vi "Finish.vi"   [LabVIEW 2016]
doc: "This VI is called just before exiting. It is expected to close I/O refnum, save collected data, etc."
uses:
  <vilib>/Rock Robotics/WPI/Utilities/WPI_GetSetVariantRefNum.vi
types:
  T1 = typedef "WPI_ServoDeviceRef.ctl" = cluster{"DeviceStatus":errorcluster, "PWM Channel":T2, "DeadBand":T3}
  T2 = typedef "FPGA_DIOPWMChannel.ctl" = enum8{"PWM 0", "PWM 1", "PWM 2", "PWM 3", "PWM 4", "PWM 5", "PWM 6", "PWM 7", "PWM 8", "PWM 9", "PWM MXP 0", "PWM MXP 1", "PWM MXP 2", "PWM MXP 3", "PWM MXP 4", "PWM MXP 5", "PWM MXP 6", "PWM MXP 7", "PWM MXP 8", "PWM MXP 9", "Invalid"}
  T3 = typedef "WPI_PWMDeadband.ctl" = cluster{"Name":string, "maxPositivePwm":i32, "minPositivePwm":i32, "centerPwm":i32, "maxNegativePwm":i32, "minNegativePwm":i32, "angularRange":u16}
  T4 = typedef "WPI_SolenoidDevRef.ctl" = cluster{"DevStatus":errorcluster, "Pneumatics Control Module":u8, "Forward Solenoid Channel":T5, "Reverse Solenoid Channel":T5}
  T5 = typedef "WPI_SolenoidChannel.ctl" = enum8{"Solenoid 0", "Solenoid 1", "Solenoid 2", "Solenoid 3", "Solenoid 4", "Solenoid 5", "Solenoid 6", "Solenoid 7", "Invalid"}
  T6 = typedef "WPI_CompressorDevRef.ctl" = cluster{"DevStatus":errorcluster, "Pneumatics Control Module":u8}
  T7 = typedef "WPI_RobotDriveDevRef.ctl" = cluster{"DevStatus":errorcluster, "Motors[]":T8[], "Square Inputs":bool, "Max Output":dbl}
  T8 = typedef "WPI_MotorControlDeviceRef.ctl" = cluster{"DeviceStatus":errorcluster, "Type":T9, "PWM":cluster{"PWM Channel":T2, "DeadBand":T3}, "CAN":cluster{"Device Number":u8, "SetOutput VI Ref":variant, "GetOutput VI Ref":variant, "Enable VI Ref":variant, "Disable VI Ref":variant, "Data":variant}, "Invert":bool}
  T9 = typedef "WPI_MotorControlType.ctl" = enum16{"PWM", "CAN"}
  T10 = typedef "WPI_JoystickDevRef.ctl" = cluster{"Device":T11}
  T11 = typedef "WPI_JoystickDeviceEnum.ctl" = enum16{"USB 0", "USB 1", "USB 2", "USB 3", "USB 4", "USB 5"}
  T12 = typedef "WPI_EncoderDevRef.ctl" = cluster{"DevStatus":errorcluster, "EncoderIndex":T13, "CounterIndex":T14, "DistancePerCount":dbl, "Decoding Type":T15}
  T13 = typedef "FPGA_EncoderIdx.ctl" = enum8{"Enc 0", "Enc 1", "Enc 2", "Enc 3", "Enc 4", "Enc 5", "Enc 6", "Enc 7", "Invalid"}
  T14 = typedef "FPGA_CounterCtrSystemIndex.ctl" = enum8{"Ctr 0", "Ctr 1", "Ctr 2", "Ctr 3", "Ctr 4", "Ctr 5", "Ctr 6", "Ctr 7", "Invalid"}
  T15 = typedef "WPI_EncoderType.ctl" = enum16{"1x", "2x", "4x"}
  T16 = typedef "WPI_AnalogChannelDevRef.ctl" = cluster{"DevStatus":errorcluster, "Analog Channel":T17}
  T17 = typedef "FPGA_AIChannel.ctl" = enum8{"AI 0", "AI 1", "AI 2", "AI 3", "AI MXP 0", "AI MXP 1", "AI MXP 2", "AI MXP 3", "Invalid"}
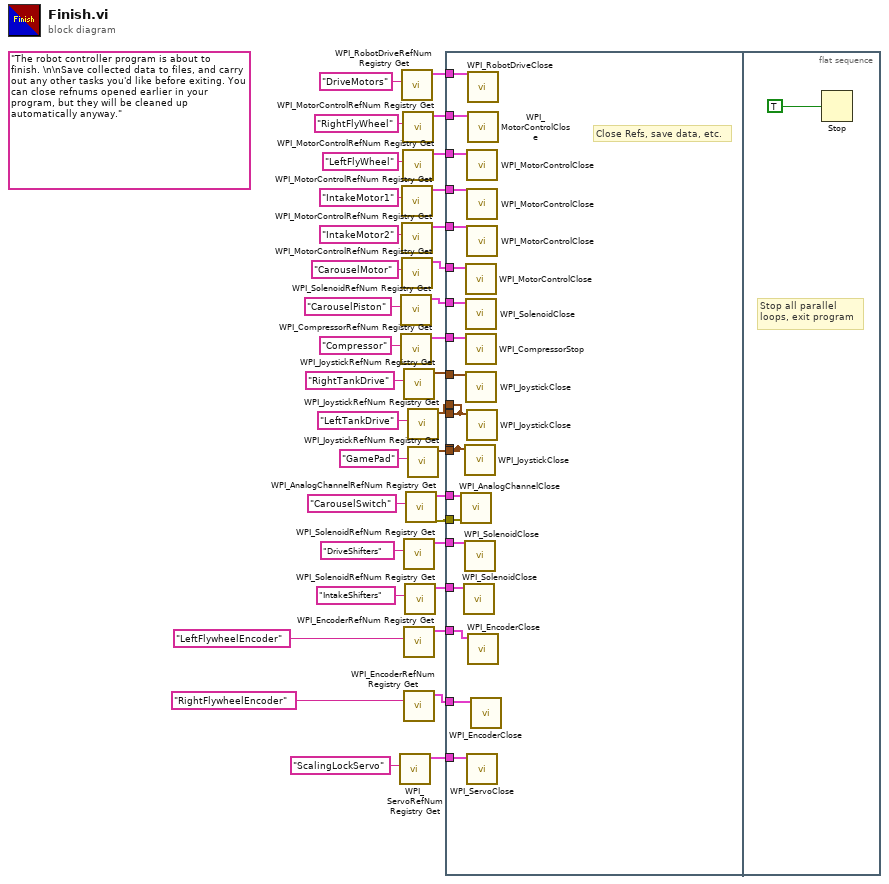
[diagram p0: block diagram]
diagram:
  (unwired) "The robot controller program is about to finish. \n\nSave collected data to files, and carry out any other tasks you'd like before exiting. You can close refnums opened earlier in your program, but they will be cleaned up automatically anyway."
  n1 = call <vilib>:"WPI_ServoRefNum Registry Get.vi"("refnum name"="ScalingLockServo") -> ("ServoDeviceRef"=w2:T1)  [unwired: 9 in, 1 out]
  n2 = call <vilib>:"WPI_SolenoidRefNum Registry Get.vi"("refnum name"="CarouselPiston") -> ("SolenoidDevRef"=w22:T4)  [unwired: 9 in, 1 out]
  n3 = call <vilib>:"WPI_CompressorRefNum Registry Get.vi"("refnum name"="Compressor") -> ("CompressorDevRef"=w21:T6)  [unwired: 9 in, 1 out]
  n4 = call <vilib>:"WPI_RobotDriveRefNum Registry Get.vi"("refnum name"="DriveMotors") -> ("RobotDriveDevRef"=w35:T7)  [unwired: 9 in, 1 out]
  n5 = call <vilib>:"WPI_MotorControlRefNum Registry Get.vi"("refnum name"="IntakeMotor1") -> ("MotorControlDevRef"=w26:T8)  [unwired: 9 in, 1 out]
  n6 = call <vilib>:"WPI_MotorControlRefNum Registry Get.vi"("refnum name"="IntakeMotor2") -> ("MotorControlDevRef"=w25:T8)  [unwired: 9 in, 1 out]
  n7 = call <vilib>:"WPI_MotorControlRefNum Registry Get.vi"("refnum name"="CarouselMotor") -> ("MotorControlDevRef"=w24:T8)  [unwired: 9 in, 1 out]
  n8 = call <vilib>:"WPI_MotorControlRefNum Registry Get.vi"("refnum name"="RightFlyWheel") -> ("MotorControlDevRef"=w28:T8)  [unwired: 9 in, 1 out]
  n9 = call <vilib>:"WPI_MotorControlRefNum Registry Get.vi"("refnum name"="LeftFlyWheel") -> ("MotorControlDevRef"=w27:T8)  [unwired: 9 in, 1 out]
  n10 = call <vilib>:"WPI_JoystickRefNum Registry Get.vi"("refnum name"="RightTankDrive") -> ("JoystickDevRef"=w19:T10)  [unwired: 9 in, 1 out]
  n11 = call <vilib>:"WPI_SolenoidRefNum Registry Get.vi"("refnum name"="DriveShifters") -> ("SolenoidDevRef"=w10:T4)  [unwired: 9 in, 1 out]
  n12 = call <vilib>:"WPI_EncoderRefNum Registry Get.vi"("refnum name"="LeftFlywheelEncoder") -> ("EncoderDevRef"=w3:T12)  [unwired: 9 in, 1 out]
  n13 = call <vilib>:"WPI_EncoderRefNum Registry Get.vi"("refnum name"="RightFlywheelEncoder") -> ("EncoderDevRef"=w4:T12)  [unwired: 9 in, 1 out]
  n14 = call <vilib>:"WPI_SolenoidRefNum Registry Get.vi"("refnum name"="IntakeShifters") -> ("SolenoidDevRef"=w9:T4)  [unwired: 9 in, 1 out]
  n15 = call <vilib>:"WPI_AnalogChannelRefNum Registry Get.vi"("refnum name"="CarouselSwitch") -> ("error out"=w12:errorcluster, "AIDeviceRef"=w11:T16)  [unwired: 9 in]
  n16 = call <vilib>:"WPI_JoystickRefNum Registry Get.vi"("refnum name"="LeftTankDrive") -> ("JoystickDevRef"=w18:T10)  [unwired: 9 in, 1 out]
  n17 = call <vilib>:"WPI_JoystickRefNum Registry Get.vi"("refnum name"="GamePad") -> ("JoystickDevRef"=w17:T10)  [unwired: 9 in, 1 out]
  n18 = flat-sequence {
    tunnel: w35 -> [w53]
    tunnel: w28 -> [w52]
    tunnel: w27 -> [w51]
    tunnel: w26 -> [w50]
    tunnel: w25 -> [w49]
    tunnel: w24 -> [w48]
    tunnel: w22 -> [w47]
    tunnel: w21 -> [w46]
    tunnel: w19 -> [w45]
    tunnel: [w44] -> _
    tunnel: [w43] -> _
    tunnel: w18 -> [w44]
    tunnel: w17 -> [w43]
    tunnel: w12 -> [w42]
    tunnel: w11 -> [w41]
    tunnel: w10 -> [w40]
    tunnel: w9 -> [w39]
    tunnel: w4 -> [w38]
    tunnel: w3 -> [w37]
    tunnel: w2 -> [w36]
    frame #0 {
      # "Close Refs, save data, etc."
      n19 = call <vilib>:"WPI_AnalogChannelClose.vi"("error in (no error)"=w42, "AIDeviceRef"=w41) -> ()  [unwired: 9 in, 1 out]
      n20 = call <vilib>:"WPI_SolenoidClose.vi"("SolenoidDevRef"=w39) -> ()  [unwired: 10 in, 1 out]
      n21 = call <vilib>:"WPI_JoystickClose.vi"("JoystickDevRef"=w43) -> ()  [unwired: 11 in]
      n22 = call <vilib>:"WPI_SolenoidClose.vi"("SolenoidDevRef"=w40) -> ()  [unwired: 10 in, 1 out]
      n23 = call <vilib>:"WPI_MotorControlClose.vi"("MotorControlDevRef"=w48) -> ()  [unwired: 10 in, 1 out]
      n24 = call <vilib>:"WPI_SolenoidClose.vi"("SolenoidDevRef"=w47) -> ()  [unwired: 10 in, 1 out]
      n25 = call <vilib>:"WPI_CompressorStop.vi"("CompressorDevRef"=w46) -> ()  [unwired: 9 in, 2 out]
      n26 = call <vilib>:"WPI_JoystickClose.vi"("JoystickDevRef"=w45) -> ()  [unwired: 11 in]
      n27 = call <vilib>:"WPI_MotorControlClose.vi"("MotorControlDevRef"=w51) -> ()  [unwired: 10 in, 1 out]
      n28 = call <vilib>:"WPI_MotorControlClose.vi"("MotorControlDevRef"=w50) -> ()  [unwired: 10 in, 1 out]
      n29 = call <vilib>:"WPI_MotorControlClose.vi"("MotorControlDevRef"=w49) -> ()  [unwired: 10 in, 1 out]
      n30 = call <vilib>:"WPI_JoystickClose.vi"("JoystickDevRef"=w44) -> ()  [unwired: 11 in]
      n31 = call <vilib>:"WPI_ServoClose.vi"("ServoDeviceRef"=w36) -> ()  [unwired: 10 in, 1 out]
      n32 = call <vilib>:"WPI_RobotDriveClose.vi"("RobotDriveDevRef"=w53) -> ()  [unwired: 10 in, 1 out]
      n33 = call <vilib>:"WPI_MotorControlClose.vi"("MotorControlDevRef"=w52) -> ()  [unwired: 10 in, 1 out]
      n34 = call <vilib>:"WPI_EncoderClose.vi"("EncoderDevRef"=w37) -> ()  [unwired: 10 in, 1 out]
      n35 = call <vilib>:"WPI_EncoderClose.vi"("EncoderDevRef"=w38) -> ()  [unwired: 10 in, 1 out]
    }
    frame #1 {
      # "Stop all parallel\nloops, exit program"
      n36 = Stop(stop? (T)=TRUE ("Quit")) -> ()
    }
  }
